vi "BREAKDOWN_FOR_DAYWISE_FINAL.vi"(6 "error in (no error)":errorcluster, 8 "To":timestamp format="%<%Y-%m-%d>T", 9 "Form":timestamp format="%<%Y-%m-%d>T", 10 "Shift":string(combo)="ALL", 11 "Select Line 2":string(combo)="ST 1") -> (0 "String":string, 1 "All Station String":string[](array[string]), 2 "condition":string, 3 "x .and. y?":bool, 4 "error out":errorcluster)   [LabVIEW 2017]
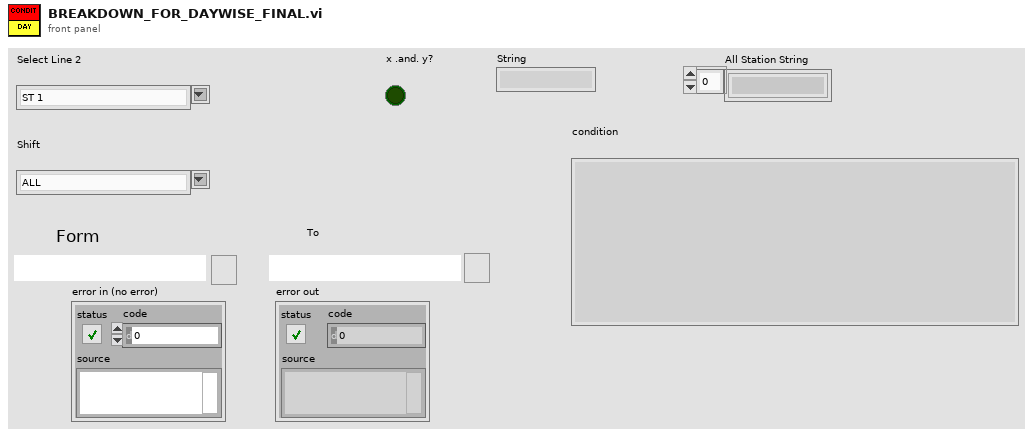
[diagram p1: front panel]
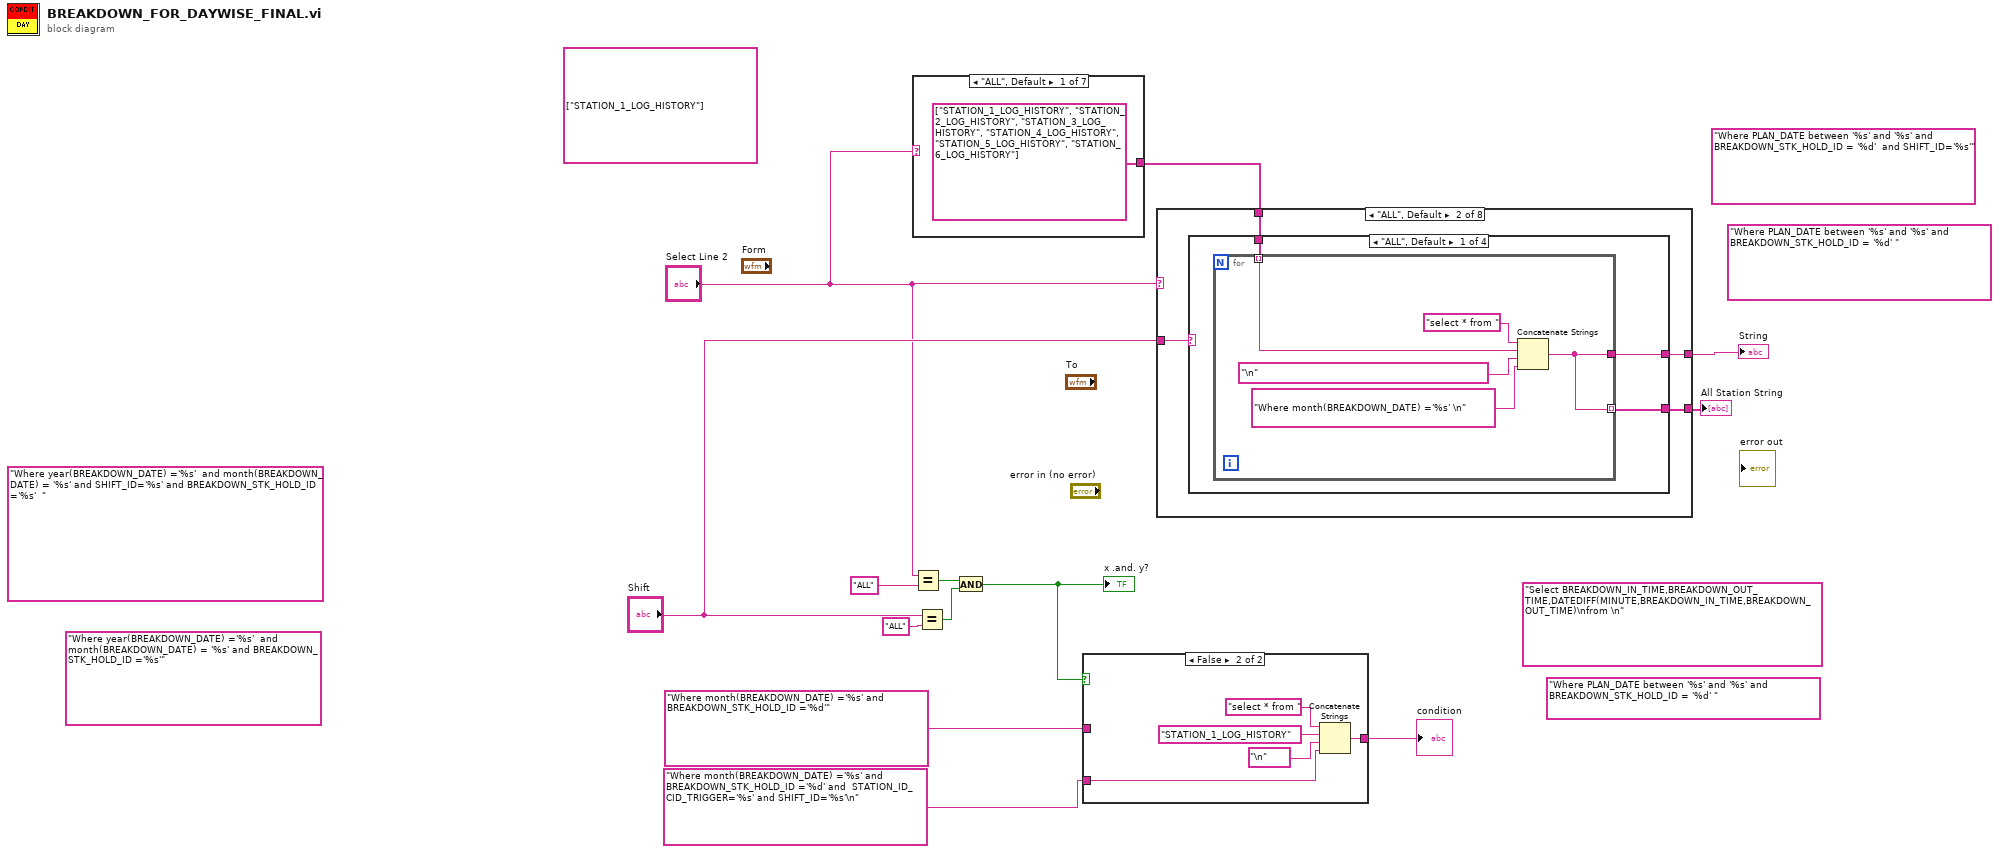
[diagram p0: block diagram]
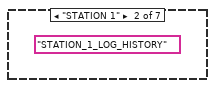
[diagram p2: hidden frame]
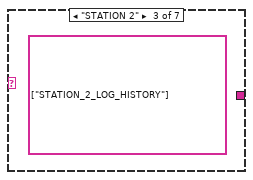
[diagram p3: hidden frame]
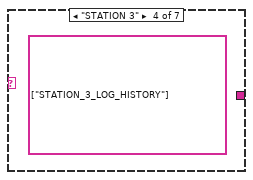
[diagram p4: hidden frame]
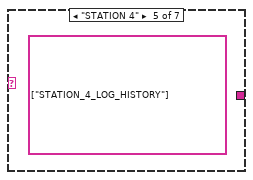
[diagram p5: hidden frame]
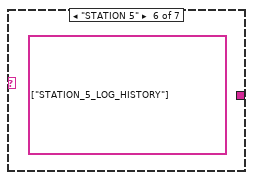
[diagram p6: hidden frame]
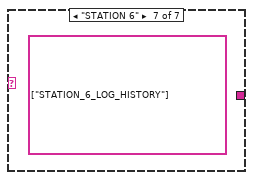
[diagram p7: hidden frame]
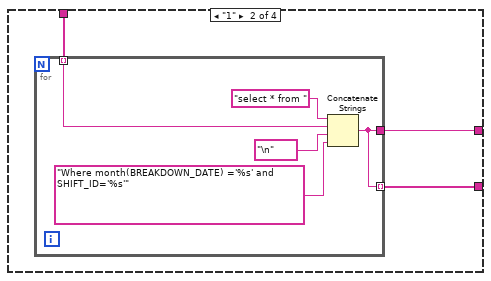
[diagram p9: hidden frame]
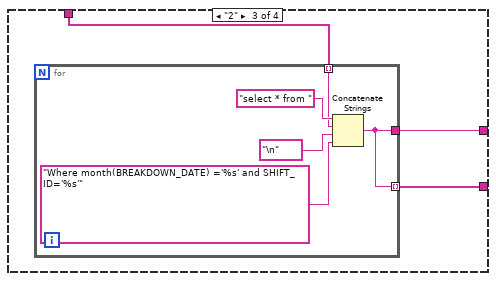
[diagram p10: hidden frame]
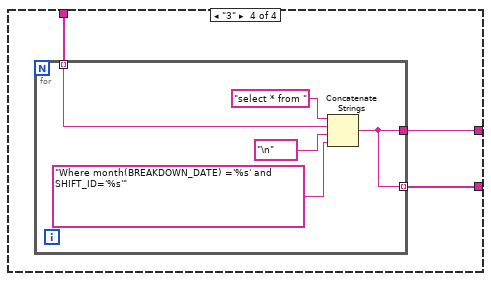
[diagram p11: hidden frame]
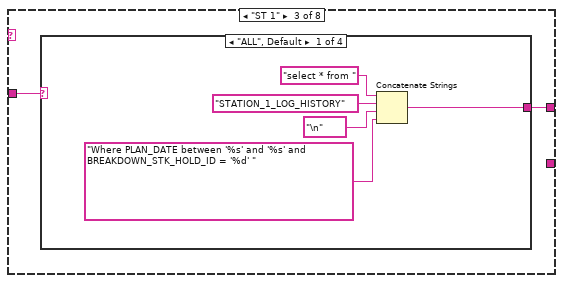
[diagram p12: hidden frame]
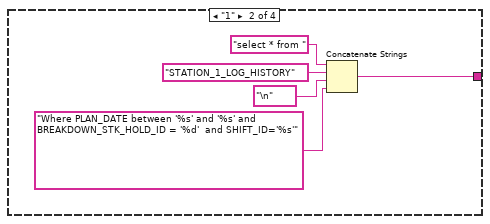
[diagram p13: hidden frame]
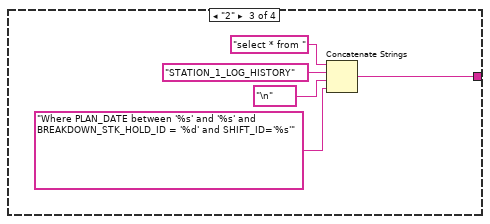
[diagram p14: hidden frame]
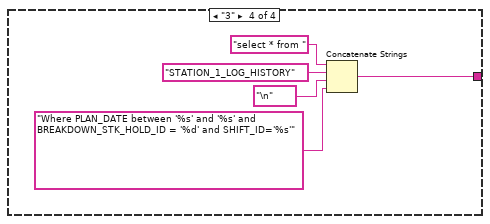
[diagram p15: hidden frame]
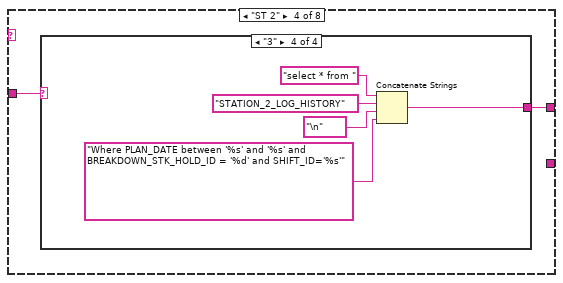
[diagram p16: hidden frame]
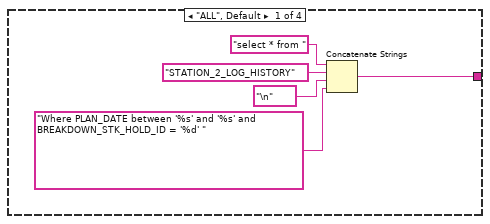
[diagram p17: hidden frame]
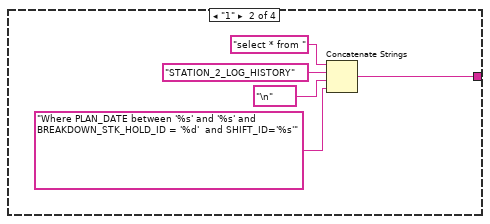
[diagram p18: hidden frame]
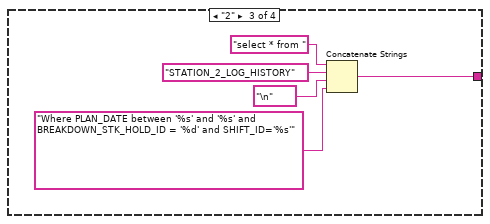
[diagram p19: hidden frame]
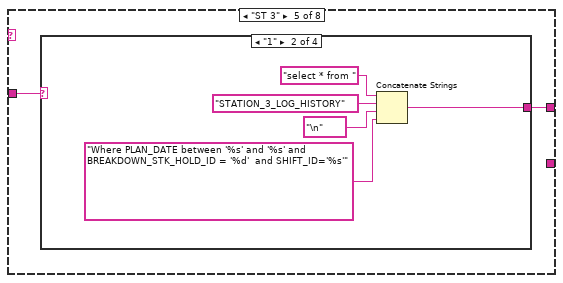
[diagram p20: hidden frame]
diagram:
  (unwired) "Where PLAN_DATE between '%s' and '%s' and BREAKDOWN_STK_HOLD_ID = '%d' " ("condition")
  (unwired) "Where PLAN_DATE between '%s' and '%s' and BREAKDOWN_STK_HOLD_ID = '%d'  and SHIFT_ID='%s'" ("condition")
  (unwired) "Where PLAN_DATE between '%s' and '%s' and BREAKDOWN_STK_HOLD_ID = '%d' "
  (unwired) "Select BREAKDOWN_IN_TIME,BREAKDOWN_OUT_TIME,DATEDIFF(MINUTE,BREAKDOWN_IN_TIME,BREAKDOWN_OUT_TIME)\nfrom \n" ("string")
  (unwired) string[] ["STATION_1_LOG_HISTORY"]
  (unwired) "Where year(BREAKDOWN_DATE) ='%s'  and month(BREAKDOWN_DATE) = '%s' and BREAKDOWN_STK_HOLD_ID ='%s'" ("condition")
  (unwired) "Where year(BREAKDOWN_DATE) ='%s'  and month(BREAKDOWN_DATE) = '%s' and SHIFT_ID='%s' and BREAKDOWN_STK_HOLD_ID ='%s'  " ("condition")
  n1 = case shown="\"ALL\", Default" "Select Line 2" {
    tunnel: [string[] ["STATION_1_LOG_HISTORY", "STATION_2_LOG_HISTORY", "STATION_3_LOG_HISTORY", "STATION_4_LOG_HISTORY", "STATION_5_LOG_HISTORY", "STATION_6_LOG_HISTORY"] _ _ _ _ _ _] -> w2
    frame "ALL", Default {
    }
    frame "STATION 1" {
      (unwired) "STATION_1_LOG_HISTORY"
    }
    frame "STATION 2" {
      (unwired) string[] ["STATION_2_LOG_HISTORY"]
    }
    frame "STATION 3" {
      (unwired) string[] ["STATION_3_LOG_HISTORY"]
    }
    frame "STATION 4" {
      (unwired) string[] ["STATION_4_LOG_HISTORY"]
    }
    frame "STATION 5" {
      (unwired) string[] ["STATION_5_LOG_HISTORY"]
    }
    frame "STATION 6" {
      (unwired) string[] ["STATION_6_LOG_HISTORY"]
    }
  }
  n2 = Equal?(x="Select Line 2", y="ALL") -> (x = y?=w11:bool)
  n3 = Equal?(x="Shift", y="ALL") -> (x = y?=w10:bool)
  n4 = And(x=w11, y=w10) -> (x .and. y?=w9:bool)
  "x .and. y?" <- w9
  n5 = case shown="False" w9 {
    tunnel: "Where month(BREAKDOWN_DATE) ='%s' and  BREAKDOWN_STK_HOLD_ID ='%d' and  STATION_ID_CID_TRIGGER='%s' and SHIFT_ID='%s'\n" ("condition") -> [_ w21]
    tunnel: "Where month(BREAKDOWN_DATE) ='%s' and  BREAKDOWN_STK_HOLD_ID ='%d'" ("condition") -> [w16 _]
    tunnel: [w15 w20] -> w6
    frame True {
      n6 = Concatenate Strings("select * from " ("string"), "STATION_1_LOG_HISTORY" ("table"), "\n" ("string"), w16) -> (w15:string)
    }
    frame False {
      n7 = Concatenate Strings("select * from " ("string"), "STATION_1_LOG_HISTORY" ("table"), "\n" ("string"), w21) -> (w20:string)
    }
  }
  "condition" <- w6
  n8 = case shown="\"ALL\", Default" "Select Line 2" {
    tunnel: "Shift" -> [_ w28 w62 w84 w106 w128 w150 w172]
    tunnel: [_ w27 w61 w83 w105 w127 w149 w171] -> w4
    tunnel: w2 -> [_ w26 _ _ _ _ _ _]
    tunnel: [_ w25 _ _ _ _ _ _] -> w1
    frame "False" {
    }
    frame "ALL", Default {
      n9 = case shown="\"ALL\", Default" w28 {
        tunnel: [w31 w39 w47 w55] -> w27
        tunnel: w26 -> [w30 w38 w46 w54]
        tunnel: [w29 w37 w45 w53] -> w25
        frame "ALL", Default {
          n10 = for {
            tunnel: [w32] -> w31
            tunnel: w30 -> [w33] mode=indexing
            tunnel: [w32] -> w29 mode=indexing
            n11 = Concatenate Strings("select * from " ("string"), w33, "\n" ("string"), "Where month(BREAKDOWN_DATE) ='%s' \n" ("condition")) -> (w32:string)
          }
        }
        frame "1" {
          n12 = for {
            tunnel: [w40] -> w39
            tunnel: w38 -> [w41] mode=indexing
            tunnel: [w40] -> w37 mode=indexing
            n13 = Concatenate Strings("select * from " ("string"), w41, "\n" ("string"), "Where month(BREAKDOWN_DATE) ='%s' and SHIFT_ID='%s'" ("condition")) -> (w40:string)
          }
        }
        frame "2" {
          n14 = for {
            tunnel: [w48] -> w47
            tunnel: w46 -> [w49] mode=indexing
            tunnel: [w48] -> w45 mode=indexing
            n15 = Concatenate Strings("select * from " ("string"), w49, "\n" ("string"), "Where month(BREAKDOWN_DATE) ='%s' and SHIFT_ID='%s'" ("condition")) -> (w48:string)
          }
        }
        frame "3" {
          n16 = for {
            tunnel: [w56] -> w55
            tunnel: w54 -> [w57] mode=indexing
            tunnel: [w56] -> w53 mode=indexing
            n17 = Concatenate Strings("select * from " ("string"), w57, "\n" ("string"), "Where month(BREAKDOWN_DATE) ='%s' and SHIFT_ID='%s'" ("condition")) -> (w56:string)
          }
        }
      }
    }
    frame "ST 1" {
      n18 = case shown="\"ALL\", Default" w62 {
        tunnel: [w63 w68 w73 w78] -> w61
        frame "ALL", Default {
          n19 = Concatenate Strings("select * from " ("string"), "STATION_1_LOG_HISTORY" ("table"), "\n" ("string"), "Where PLAN_DATE between '%s' and '%s' and BREAKDOWN_STK_HOLD_ID = '%d' " ("condition")) -> (w63:string)
        }
        frame "1" {
          n20 = Concatenate Strings("select * from " ("string"), "STATION_1_LOG_HISTORY" ("table"), "\n" ("string"), "Where PLAN_DATE between '%s' and '%s' and BREAKDOWN_STK_HOLD_ID = '%d'  and SHIFT_ID='%s'" ("condition")) -> (w68:string)
        }
        frame "2" {
          n21 = Concatenate Strings("select * from " ("string"), "STATION_1_LOG_HISTORY" ("table"), "\n" ("string"), "Where PLAN_DATE between '%s' and '%s' and BREAKDOWN_STK_HOLD_ID = '%d' and SHIFT_ID='%s'" ("condition")) -> (w73:string)
        }
        frame "3" {
          n22 = Concatenate Strings("select * from " ("string"), "STATION_1_LOG_HISTORY" ("table"), "\n" ("string"), "Where PLAN_DATE between '%s' and '%s' and BREAKDOWN_STK_HOLD_ID = '%d' and SHIFT_ID='%s'" ("condition")) -> (w78:string)
        }
      }
    }
    frame "ST 2" {
      n23 = case shown="\"3\"" w84 {
        tunnel: [w85 w90 w95 w100] -> w83
        frame "ALL", Default {
          n24 = Concatenate Strings("select * from " ("string"), "STATION_2_LOG_HISTORY" ("table"), "\n" ("string"), "Where PLAN_DATE between '%s' and '%s' and BREAKDOWN_STK_HOLD_ID = '%d' " ("condition")) -> (w85:string)
        }
        frame "1" {
          n25 = Concatenate Strings("select * from " ("string"), "STATION_2_LOG_HISTORY" ("table"), "\n" ("string"), "Where PLAN_DATE between '%s' and '%s' and BREAKDOWN_STK_HOLD_ID = '%d'  and SHIFT_ID='%s'" ("condition")) -> (w90:string)
        }
        frame "2" {
          n26 = Concatenate Strings("select * from " ("string"), "STATION_2_LOG_HISTORY" ("table"), "\n" ("string"), "Where PLAN_DATE between '%s' and '%s' and BREAKDOWN_STK_HOLD_ID = '%d' and SHIFT_ID='%s'" ("condition")) -> (w95:string)
        }
        frame "3" {
          n27 = Concatenate Strings("select * from " ("string"), "STATION_2_LOG_HISTORY" ("table"), "\n" ("string"), "Where PLAN_DATE between '%s' and '%s' and BREAKDOWN_STK_HOLD_ID = '%d' and SHIFT_ID='%s'" ("condition")) -> (w100:string)
        }
      }
    }
    frame "ST 3" {
      n28 = case shown="\"1\"" w106 {
        tunnel: [w107 w112 w117 w122] -> w105
        frame "ALL", Default {
          n29 = Concatenate Strings("select * from " ("string"), "STATION_3_LOG_HISTORY" ("table"), "\n" ("string"), "Where PLAN_DATE between '%s' and '%s' and BREAKDOWN_STK_HOLD_ID = '%d' " ("condition")) -> (w107:string)
        }
        frame "1" {
          n30 = Concatenate Strings("select * from " ("string"), "STATION_3_LOG_HISTORY" ("table"), "\n" ("string"), "Where PLAN_DATE between '%s' and '%s' and BREAKDOWN_STK_HOLD_ID = '%d'  and SHIFT_ID='%s'" ("condition")) -> (w112:string)
        }
        frame "2" {
          n31 = Concatenate Strings("select * from " ("string"), "STATION_3_LOG_HISTORY" ("table"), "\n" ("string"), "Where PLAN_DATE between '%s' and '%s' and BREAKDOWN_STK_HOLD_ID = '%d' and SHIFT_ID='%s'" ("condition")) -> (w117:string)
        }
        frame "3" {
          n32 = Concatenate Strings("select * from " ("string"), "STATION_3_LOG_HISTORY" ("table"), "\n" ("string"), "Where PLAN_DATE between '%s' and '%s' and BREAKDOWN_STK_HOLD_ID = '%d' and SHIFT_ID='%s'" ("condition")) -> (w122:string)
        }
      }
    }
    frame "ST 4" {
      n33 = case shown="\"ALL\", Default" w128 {
        tunnel: [w129 w134 w139 w144] -> w127
        frame "ALL", Default {
          n34 = Concatenate Strings("select * from " ("string"), "STATION_4_LOG_HISTORY" ("table"), "\n" ("string"), "Where PLAN_DATE between '%s' and '%s' and BREAKDOWN_STK_HOLD_ID = '%d' " ("condition")) -> (w129:string)
        }
        frame "1" {
          n35 = Concatenate Strings("select * from " ("string"), "STATION_4_LOG_HISTORY" ("table"), "\n" ("string"), "Where PLAN_DATE between '%s' and '%s' and BREAKDOWN_STK_HOLD_ID = '%d'  and SHIFT_ID='%s'" ("condition")) -> (w134:string)
        }
        frame "2" {
          n36 = Concatenate Strings("select * from " ("string"), "STATION_4_LOG_HISTORY" ("table"), "\n" ("string"), "Where PLAN_DATE between '%s' and '%s' and BREAKDOWN_STK_HOLD_ID = '%d' and SHIFT_ID='%s'" ("condition")) -> (w139:string)
        }
        frame "3" {
          n37 = Concatenate Strings("select * from " ("string"), "STATION_4_LOG_HISTORY" ("table"), "\n" ("string"), "Where PLAN_DATE between '%s' and '%s' and BREAKDOWN_STK_HOLD_ID = '%d' and SHIFT_ID='%s'" ("condition")) -> (w144:string)
        }
      }
    }
    frame "ST 5" {
      n38 = case shown="\"1\"" w150 {
        tunnel: [w151 w156 w161 w166] -> w149
        frame "ALL", Default {
          n39 = Concatenate Strings("select * from " ("string"), "STATION_5_LOG_HISTORY" ("table"), "\n" ("string"), "Where PLAN_DATE between '%s' and '%s' and BREAKDOWN_STK_HOLD_ID = '%d' " ("condition")) -> (w151:string)
        }
        frame "1" {
          n40 = Concatenate Strings("select * from " ("string"), "STATION_5_LOG_HISTORY" ("table"), "\n" ("string"), "Where PLAN_DATE between '%s' and '%s' and BREAKDOWN_STK_HOLD_ID = '%d'  and SHIFT_ID='%s'" ("condition")) -> (w156:string)
        }
        frame "2" {
          n41 = Concatenate Strings("select * from " ("string"), "STATION_5_LOG_HISTORY" ("table"), "\n" ("string"), "Where PLAN_DATE between '%s' and '%s' and BREAKDOWN_STK_HOLD_ID = '%d' and SHIFT_ID='%s'" ("condition")) -> (w161:string)
        }
        frame "3" {
          n42 = Concatenate Strings("select * from " ("string"), "STATION_5_LOG_HISTORY" ("table"), "\n" ("string"), "Where PLAN_DATE between '%s' and '%s' and BREAKDOWN_STK_HOLD_ID = '%d' and SHIFT_ID='%s'" ("condition")) -> (w166:string)
        }
      }
    }
    frame "ST 6" {
      n43 = case shown="\"ALL\", Default" w172 {
        tunnel: [w173 w178 w183 w188] -> w171
        frame "ALL", Default {
          n44 = Concatenate Strings("select * from " ("string"), "STATION_6_LOG_HISTORY" ("table"), "\n" ("string"), "Where PLAN_DATE between '%s' and '%s' and BREAKDOWN_STK_HOLD_ID = '%d' " ("condition")) -> (w173:string)
        }
        frame "1" {
          n45 = Concatenate Strings("select * from " ("string"), "STATION_6_LOG_HISTORY" ("table"), "\n" ("string"), "Where PLAN_DATE between '%s' and '%s' and BREAKDOWN_STK_HOLD_ID = '%d'  and SHIFT_ID='%s'" ("condition")) -> (w178:string)
        }
        frame "2" {
          n46 = Concatenate Strings("select * from " ("string"), "STATION_6_LOG_HISTORY" ("table"), "\n" ("string"), "Where PLAN_DATE between '%s' and '%s' and BREAKDOWN_STK_HOLD_ID = '%d' and SHIFT_ID='%s'" ("condition")) -> (w183:string)
        }
        frame "3" {
          n47 = Concatenate Strings("select * from " ("string"), "STATION_6_LOG_HISTORY" ("table"), "\n" ("string"), "Where PLAN_DATE between '%s' and '%s' and BREAKDOWN_STK_HOLD_ID = '%d' and SHIFT_ID='%s'" ("condition")) -> (w188:string)
        }
      }
    }
  }
  "String" <- w4
  "All Station String" <- w1
